vi "Host to Target.vi"(11 "Ready for Input":bool) -> (2 "Output Valid":bool, 3 "Data":u32)   [LabVIEW 2015]
uses:
  <vilib>/rvi/interface/RandomDataEmulation/niFpgaRandomDataHandleErrors.vi
  <vilib>/rvi/DataTransferAndStorage/Container/XNode/niFpgaContainer.xnode
  <vilib>/rvi/interface/RandomDataEmulation/nirviRandomDataFpgaReadWriteTemplate.vi
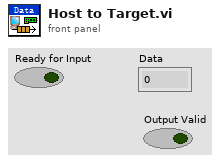
[diagram p1: front panel]
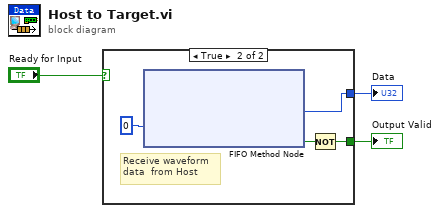
[diagram p0: block diagram]
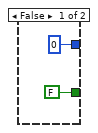
[diagram p2: hidden frame]
diagram:
  n1 = case shown="True" "Ready for Input" {
    tunnel: [FALSE w7] -> w3
    tunnel: [u32 0 ("Element") w6] -> w2
    frame False {
    }
    frame True {
      # "Receive waveform\ndata  from Host"
      n2 = xnode ("FIFO Method Node")("Timeout"=0) -> ("Element"=w6:u32, "Timed Out?"=w8:bool)  [unwired: 1 in, 1 out]
      n3 = Not(x=w8) -> (.not. x?=w7:bool)
    }
  }
  "Output Valid" <- w3
  "Data" <- w2
